vi "SubVI_Color.vi"() -> (0 "電阻值 1":u32(colorbox), 1 "電阻值 2":u32(colorbox), 3 "R1":i32, 4 "R2":i32, 5 "電阻值 3":u32(colorbox), 6 "電阻誤差":u32(colorbox), 8 "R3":i32, 9 "R_error":i32)   [LabVIEW 2014]
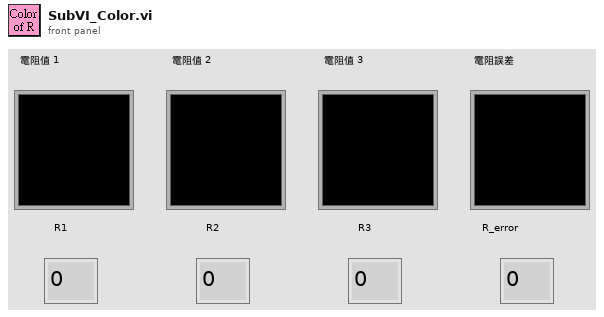
[diagram p1: front panel]
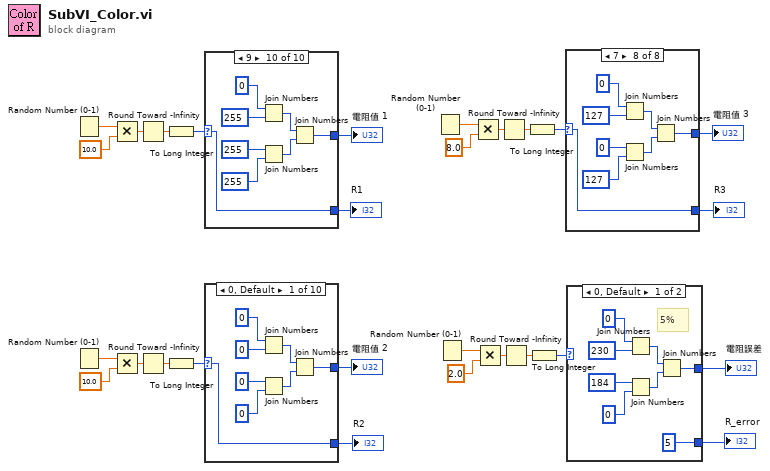
[diagram p0: block diagram]
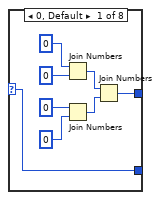
[diagram p2: hidden frame]
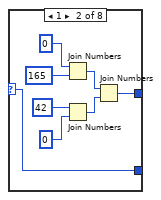
[diagram p3: hidden frame]
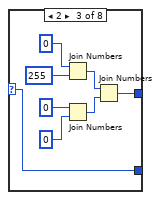
[diagram p4: hidden frame]
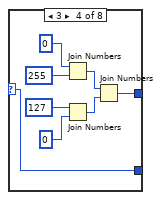
[diagram p5: hidden frame]
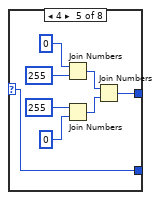
[diagram p6: hidden frame]
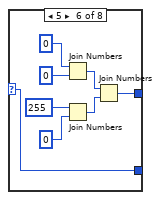
[diagram p7: hidden frame]
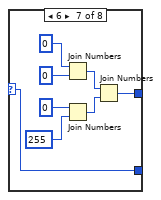
[diagram p8: hidden frame]
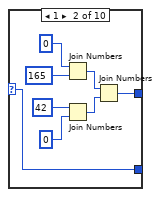
[diagram p9: hidden frame]
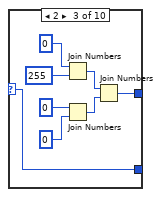
[diagram p10: hidden frame]
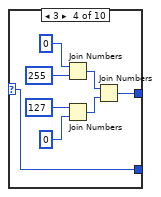
[diagram p11: hidden frame]
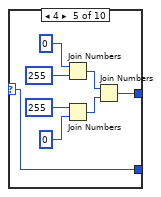
[diagram p12: hidden frame]
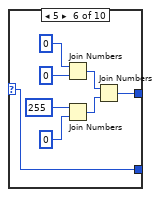
[diagram p13: hidden frame]
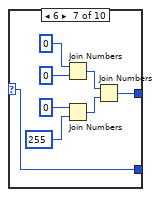
[diagram p14: hidden frame]
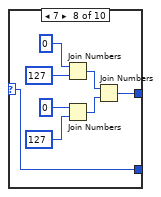
[diagram p15: hidden frame]
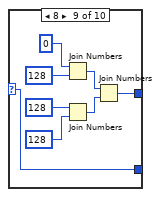
[diagram p16: hidden frame]
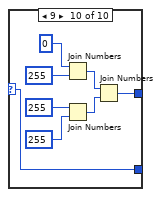
[diagram p17: hidden frame]
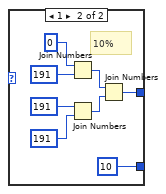
[diagram p18: hidden frame]
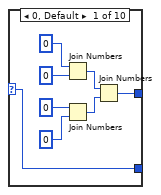
[diagram p19: hidden frame]
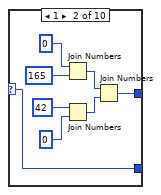
[diagram p20: hidden frame]
diagram:
  n1 = Random Number (0-1)() -> (number: 0 to 1=w28:dbl)
  n2 = Random Number (0-1)() -> (number: 0 to 1=w16:dbl)
  n3 = Multiply(x=w28, y=10.0) -> (x*y=w26:dbl)
  n4 = Multiply(x=w16, y=10.0) -> (x*y=w14:dbl)
  n5 = Round Toward -Infinity(1:w26) -> (0:w25:dbl)
  n6 = Round Toward -Infinity(1:w14) -> (0:w13:dbl)
  n7 = To Long Integer(number=w25) -> (32bit integer=w24:i32)
  n8 = To Long Integer(number=w13) -> (32bit integer=w12:i32)
  n9 = case shown="9" w24 {
    selector: w24 -> [w29 w37 w45 w53 w61 w69 w77 w85 w93 w101]
    tunnel: [w30 w38 w46 w54 w62 w70 w78 w86 w94 w102] -> w23
    tunnel: [w29 w37 w45 w53 w61 w69 w77 w85 w93 w101] -> w4
    frame 0, Default {
      n10 = Join Numbers(hi=u8 0, lo=u8 0) -> ((hi.lo)=w32:u16)
      n11 = Join Numbers(hi=u8 0, lo=u8 0) -> ((hi.lo)=w31:u16)
      n12 = Join Numbers(hi=w32, lo=w31) -> ((hi.lo)=w30:u32)
    }
    frame 1 {
      n13 = Join Numbers(hi=u8 0, lo=u8 165) -> ((hi.lo)=w40:u16)
      n14 = Join Numbers(hi=u8 42, lo=u8 0) -> ((hi.lo)=w39:u16)
      n15 = Join Numbers(hi=w40, lo=w39) -> ((hi.lo)=w38:u32)
    }
    frame 2 {
      n16 = Join Numbers(hi=u8 0, lo=u8 255) -> ((hi.lo)=w48:u16)
      n17 = Join Numbers(hi=u8 0, lo=u8 0) -> ((hi.lo)=w47:u16)
      n18 = Join Numbers(hi=w48, lo=w47) -> ((hi.lo)=w46:u32)
    }
    frame 3 {
      n19 = Join Numbers(hi=u8 0, lo=u8 255) -> ((hi.lo)=w56:u16)
      n20 = Join Numbers(hi=u8 127, lo=u8 0) -> ((hi.lo)=w55:u16)
      n21 = Join Numbers(hi=w56, lo=w55) -> ((hi.lo)=w54:u32)
    }
    frame 4 {
      n22 = Join Numbers(hi=u8 0, lo=u8 255) -> ((hi.lo)=w64:u16)
      n23 = Join Numbers(hi=u8 255, lo=u8 0) -> ((hi.lo)=w63:u16)
      n24 = Join Numbers(hi=w64, lo=w63) -> ((hi.lo)=w62:u32)
    }
    frame 5 {
      n25 = Join Numbers(hi=u8 0, lo=u8 0) -> ((hi.lo)=w72:u16)
      n26 = Join Numbers(hi=u8 255, lo=u8 0) -> ((hi.lo)=w71:u16)
      n27 = Join Numbers(hi=w72, lo=w71) -> ((hi.lo)=w70:u32)
    }
    frame 6 {
      n28 = Join Numbers(hi=u8 0, lo=u8 0) -> ((hi.lo)=w80:u16)
      n29 = Join Numbers(hi=u8 0, lo=u8 255) -> ((hi.lo)=w79:u16)
      n30 = Join Numbers(hi=w80, lo=w79) -> ((hi.lo)=w78:u32)
    }
    frame 7 {
      n31 = Join Numbers(hi=u8 0, lo=u8 127) -> ((hi.lo)=w88:u16)
      n32 = Join Numbers(hi=u8 0, lo=u8 127) -> ((hi.lo)=w87:u16)
      n33 = Join Numbers(hi=w88, lo=w87) -> ((hi.lo)=w86:u32)
    }
    frame 8 {
      n34 = Join Numbers(hi=u8 0, lo=u8 128) -> ((hi.lo)=w96:u16)
      n35 = Join Numbers(hi=u8 128, lo=u8 128) -> ((hi.lo)=w95:u16)
      n36 = Join Numbers(hi=w96, lo=w95) -> ((hi.lo)=w94:u32)
    }
    frame 9 {
      n37 = Join Numbers(hi=u8 0, lo=u8 255) -> ((hi.lo)=w104:u16)
      n38 = Join Numbers(hi=u8 255, lo=u8 255) -> ((hi.lo)=w103:u16)
      n39 = Join Numbers(hi=w104, lo=w103) -> ((hi.lo)=w102:u32)
    }
  }
  "電阻值 1" <- w23
  "R1" <- w4
  n40 = case shown="0, Default" w12 {
    selector: w12 -> [w109 w117 w125 w133 w141 w149 w157 w165 w173 w181]
    tunnel: [w110 w118 w126 w134 w142 w150 w158 w166 w174 w182] -> w11
    tunnel: [w109 w117 w125 w133 w141 w149 w157 w165 w173 w181] -> w3
    frame 0, Default {
      n41 = Join Numbers(hi=u8 0, lo=u8 0) -> ((hi.lo)=w112:u16)
      n42 = Join Numbers(hi=u8 0, lo=u8 0) -> ((hi.lo)=w111:u16)
      n43 = Join Numbers(hi=w112, lo=w111) -> ((hi.lo)=w110:u32)
    }
    frame 1 {
      n44 = Join Numbers(hi=u8 0, lo=u8 165) -> ((hi.lo)=w120:u16)
      n45 = Join Numbers(hi=u8 42, lo=u8 0) -> ((hi.lo)=w119:u16)
      n46 = Join Numbers(hi=w120, lo=w119) -> ((hi.lo)=w118:u32)
    }
    frame 2 {
      n47 = Join Numbers(hi=u8 0, lo=u8 255) -> ((hi.lo)=w128:u16)
      n48 = Join Numbers(hi=u8 0, lo=u8 0) -> ((hi.lo)=w127:u16)
      n49 = Join Numbers(hi=w128, lo=w127) -> ((hi.lo)=w126:u32)
    }
    frame 3 {
      n50 = Join Numbers(hi=u8 0, lo=u8 255) -> ((hi.lo)=w136:u16)
      n51 = Join Numbers(hi=u8 127, lo=u8 0) -> ((hi.lo)=w135:u16)
      n52 = Join Numbers(hi=w136, lo=w135) -> ((hi.lo)=w134:u32)
    }
    frame 4 {
      n53 = Join Numbers(hi=u8 0, lo=u8 255) -> ((hi.lo)=w144:u16)
      n54 = Join Numbers(hi=u8 255, lo=u8 0) -> ((hi.lo)=w143:u16)
      n55 = Join Numbers(hi=w144, lo=w143) -> ((hi.lo)=w142:u32)
    }
    frame 5 {
      n56 = Join Numbers(hi=u8 0, lo=u8 0) -> ((hi.lo)=w152:u16)
      n57 = Join Numbers(hi=u8 255, lo=u8 0) -> ((hi.lo)=w151:u16)
      n58 = Join Numbers(hi=w152, lo=w151) -> ((hi.lo)=w150:u32)
    }
    frame 6 {
      n59 = Join Numbers(hi=u8 0, lo=u8 0) -> ((hi.lo)=w160:u16)
      n60 = Join Numbers(hi=u8 0, lo=u8 255) -> ((hi.lo)=w159:u16)
      n61 = Join Numbers(hi=w160, lo=w159) -> ((hi.lo)=w158:u32)
    }
    frame 7 {
      n62 = Join Numbers(hi=u8 0, lo=u8 127) -> ((hi.lo)=w168:u16)
      n63 = Join Numbers(hi=u8 0, lo=u8 127) -> ((hi.lo)=w167:u16)
      n64 = Join Numbers(hi=w168, lo=w167) -> ((hi.lo)=w166:u32)
    }
    frame 8 {
      n65 = Join Numbers(hi=u8 0, lo=u8 128) -> ((hi.lo)=w176:u16)
      n66 = Join Numbers(hi=u8 128, lo=u8 128) -> ((hi.lo)=w175:u16)
      n67 = Join Numbers(hi=w176, lo=w175) -> ((hi.lo)=w174:u32)
    }
    frame 9 {
      n68 = Join Numbers(hi=u8 0, lo=u8 255) -> ((hi.lo)=w184:u16)
      n69 = Join Numbers(hi=u8 255, lo=u8 255) -> ((hi.lo)=w183:u16)
      n70 = Join Numbers(hi=w184, lo=w183) -> ((hi.lo)=w182:u32)
    }
  }
  "電阻值 2" <- w11
  "R2" <- w3
  n71 = Random Number (0-1)() -> (number: 0 to 1=w10:dbl)
  n72 = Random Number (0-1)() -> (number: 0 to 1=w21:dbl)
  n73 = Multiply(x=w10, y=8.0) -> (x*y=w8:dbl)
  n74 = Multiply(x=w21, y=2.0) -> (x*y=w19:dbl)
  n75 = Round Toward -Infinity(1:w8) -> (0:w7:dbl)
  n76 = Round Toward -Infinity(1:w19) -> (0:w18:dbl)
  n77 = To Long Integer(number=w7) -> (32bit integer=w6:i32)
  n78 = To Long Integer(number=w18) -> (32bit integer=w17:i32)
  n79 = case shown="7" w6 {
    selector: w6 -> [w189 w197 w205 w213 w221 w229 w237 w245]
    tunnel: [w190 w198 w206 w214 w222 w230 w238 w246] -> w5
    tunnel: [w189 w197 w205 w213 w221 w229 w237 w245] -> w2
    frame 0, Default {
      n80 = Join Numbers(hi=u8 0, lo=u8 0) -> ((hi.lo)=w192:u16)
      n81 = Join Numbers(hi=u8 0, lo=u8 0) -> ((hi.lo)=w191:u16)
      n82 = Join Numbers(hi=w192, lo=w191) -> ((hi.lo)=w190:u32)
    }
    frame 1 {
      n83 = Join Numbers(hi=u8 0, lo=u8 165) -> ((hi.lo)=w200:u16)
      n84 = Join Numbers(hi=u8 42, lo=u8 0) -> ((hi.lo)=w199:u16)
      n85 = Join Numbers(hi=w200, lo=w199) -> ((hi.lo)=w198:u32)
    }
    frame 2 {
      n86 = Join Numbers(hi=u8 0, lo=u8 255) -> ((hi.lo)=w208:u16)
      n87 = Join Numbers(hi=u8 0, lo=u8 0) -> ((hi.lo)=w207:u16)
      n88 = Join Numbers(hi=w208, lo=w207) -> ((hi.lo)=w206:u32)
    }
    frame 3 {
      n89 = Join Numbers(hi=u8 0, lo=u8 255) -> ((hi.lo)=w216:u16)
      n90 = Join Numbers(hi=u8 127, lo=u8 0) -> ((hi.lo)=w215:u16)
      n91 = Join Numbers(hi=w216, lo=w215) -> ((hi.lo)=w214:u32)
    }
    frame 4 {
      n92 = Join Numbers(hi=u8 0, lo=u8 255) -> ((hi.lo)=w224:u16)
      n93 = Join Numbers(hi=u8 255, lo=u8 0) -> ((hi.lo)=w223:u16)
      n94 = Join Numbers(hi=w224, lo=w223) -> ((hi.lo)=w222:u32)
    }
    frame 5 {
      n95 = Join Numbers(hi=u8 0, lo=u8 0) -> ((hi.lo)=w232:u16)
      n96 = Join Numbers(hi=u8 255, lo=u8 0) -> ((hi.lo)=w231:u16)
      n97 = Join Numbers(hi=w232, lo=w231) -> ((hi.lo)=w230:u32)
    }
    frame 6 {
      n98 = Join Numbers(hi=u8 0, lo=u8 0) -> ((hi.lo)=w240:u16)
      n99 = Join Numbers(hi=u8 0, lo=u8 255) -> ((hi.lo)=w239:u16)
      n100 = Join Numbers(hi=w240, lo=w239) -> ((hi.lo)=w238:u32)
    }
    frame 7 {
      n101 = Join Numbers(hi=u8 0, lo=u8 127) -> ((hi.lo)=w248:u16)
      n102 = Join Numbers(hi=u8 0, lo=u8 127) -> ((hi.lo)=w247:u16)
      n103 = Join Numbers(hi=w248, lo=w247) -> ((hi.lo)=w246:u32)
    }
  }
  "電阻值 3" <- w5
  "R3" <- w2
  n104 = case shown="0, Default" w17 {
    tunnel: [w254 w262] -> w22
    tunnel: [5 ("R error") 10 ("R error")] -> w1
    frame 0, Default {
      # "5%"
      n105 = Join Numbers(hi=u8 0, lo=u8 230) -> ((hi.lo)=w256:u16)
      n106 = Join Numbers(hi=u8 184, lo=u8 0) -> ((hi.lo)=w255:u16)
      n107 = Join Numbers(hi=w256, lo=w255) -> ((hi.lo)=w254:u32)
    }
    frame 1 {
      # "10%"
      n108 = Join Numbers(hi=u8 0, lo=u8 191) -> ((hi.lo)=w264:u16)
      n109 = Join Numbers(hi=u8 191, lo=u8 191) -> ((hi.lo)=w263:u16)
      n110 = Join Numbers(hi=w264, lo=w263) -> ((hi.lo)=w262:u32)
    }
  }
  "電阻誤差" <- w22
  "R_error" <- w1
